vi "Legalposition.vi"(0 "Chessboard":T2, 5 "ItemIndex":T1, 7 "StoneColor":u16, 11 "error in (no error)":errorcluster) -> (4 "Chessboard out":T2, 6 "ItemIndex out":T1, 8 "StoneColor out":u16, 10 "Legal?":bool, 15 "error out":errorcluster)   [LabVIEW 2009]
doc: "To judge if the position is Legal.\nLegal: Empty and can move stone on."
uses:
  Controls/Chess.ctl
  Controls/ItemIndex.ctl
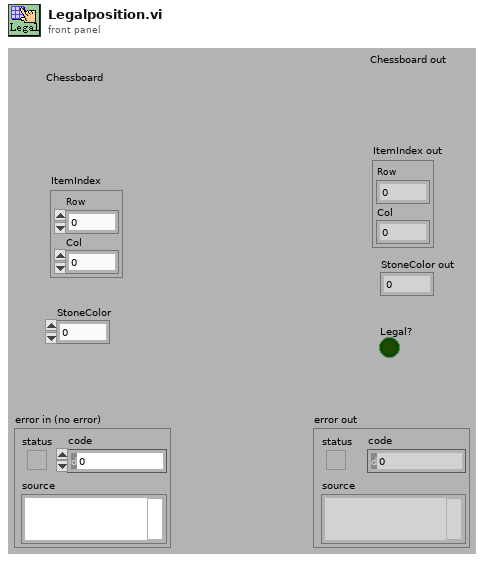
[diagram p1: front panel]
types:
  T1 = typedef "ItemIndex.ctl" = cluster{"Row":i32, "Col":i32}
  T2 = typedef "Chess.ctl" = u16[][]
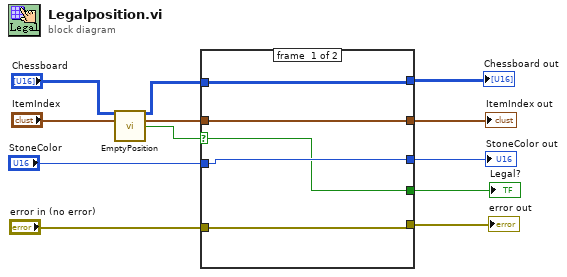
[diagram p0: block diagram]
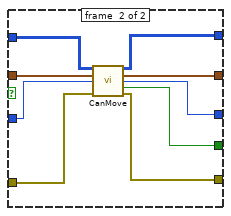
[diagram p2: hidden frame]
diagram:
  n1 = call "EmptyPosition.vi"("Chessboard in"="Chessboard", "ItemIndex"="ItemIndex") -> ("Chessboard out"=w9:T2, "ItemIndex out"=w8:T1, "EmptyPosition?"=w11:bool)  [unwired: 10 in, 1 out]
  n2 = case shown="True" w11 {
    selector: w11 -> [w14 _]
    tunnel: w9 -> [w17 w26]
    tunnel: w8 -> [w16 w25]
    tunnel: "StoneColor" -> [w15 w24]
    tunnel: "error in (no error)" -> [w13 w23]
    tunnel: [w14 w22] -> w1
    tunnel: [w17 w21] -> w5
    tunnel: [w16 w20] -> w4
    tunnel: [w15 w19] -> w3
    tunnel: [w13 w18] -> w2
    frame #0 {
    }
    frame #1 {
      n3 = call "CanMove.vi"("Chessboard in"=w26, "ItemIndex"=w25, "StoneColor"=w24, "error in (no error)"=w23) -> ("Chessboard out"=w21:T2, "ItemIndex out"=w20:T1, "StoneColor out"=w19:u16, "CanMove?"=w22:bool, "error out"=w18:errorcluster)  [unwired: 7 in]
    }
  }
  "error out" <- w2
  "Chessboard out" <- w5
  "ItemIndex out" <- w4
  "StoneColor out" <- w3
  "Legal?" <- w1
